vi "HTTPHeaderLine.vi"(8 "error in (no error)":errorcluster, 11 "HTTP Request Line":string) -> (0 "error out":errorcluster, 1 "Reason-Phrase":string, 2 "Status Code":T1 items=["Forbidden"=403, "Not Found"=0, "Upgrade Required"=426], 3 "Http Version":string)   [LabVIEW 2016, in "WebSocket Actors.lvlib" / "WebSocket Server.lvclass"]
doc: "Parses the first line of the received HTTP headers (e.g. GET / HTTP/1.1)\nWebSockets 1.6.0.22\nSam Sharp - MediaMongrels Ltd\nCopyright (c) 2016, MediaMongrels Ltd"
uses:
  WebSocket Server.lvclass
  Http Response Codes.ctl
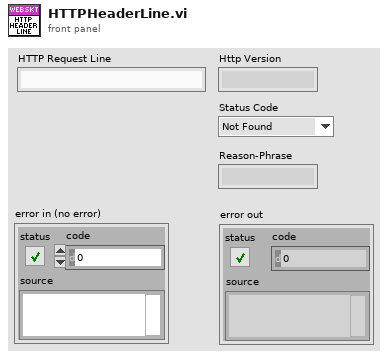
[diagram p1: front panel]
types:
  T1 = typedef "WebSocket Actors.lvlib/WebSocket Server.lvclass/Http Response Codes.ctl" = u16
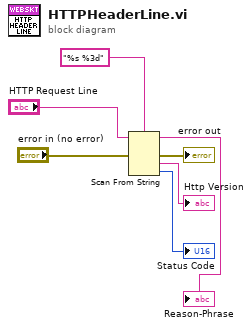
[diagram p0: block diagram]
diagram:
  n1 = Scan From String(format string="%s %3d", input string="HTTP Request Line", error in="error in (no error)") -> (remaining string=→"Reason-Phrase":string, error out=→"error out":errorcluster, output 1=→"Http Version":string, output 2=→"Status Code":T1)  [unwired: 3 in, 1 out]
